vi "Close CurrentSource.vi"(6 "Source 2":T1(ring), 8 "error in (no error)":errorcluster, 10 "task in":refnum<k24>, 11 "VISA Refnum in":refnum<visa-resource-name>) -> ()   [LabVIEW 2024]
uses:
  <instrlib>/ULx/ULx_LV.dll
  Documents/LabVIEW Data/TestHarnessDPL_v24/Program Files/National Instruments/LabVIEW 2024/instr.lib/Keithley 24XX/Keithley 24XX.lvlib
panel:
  out "error out":errorcluster
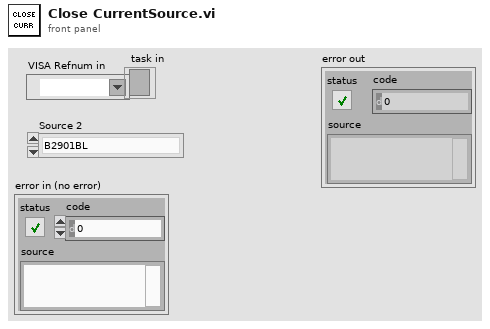
[diagram p1: front panel]
types:
  T1 = enum16{"B2901BL", "USB-3104 10M o/p3", "USB-3104 100K o/p5"}
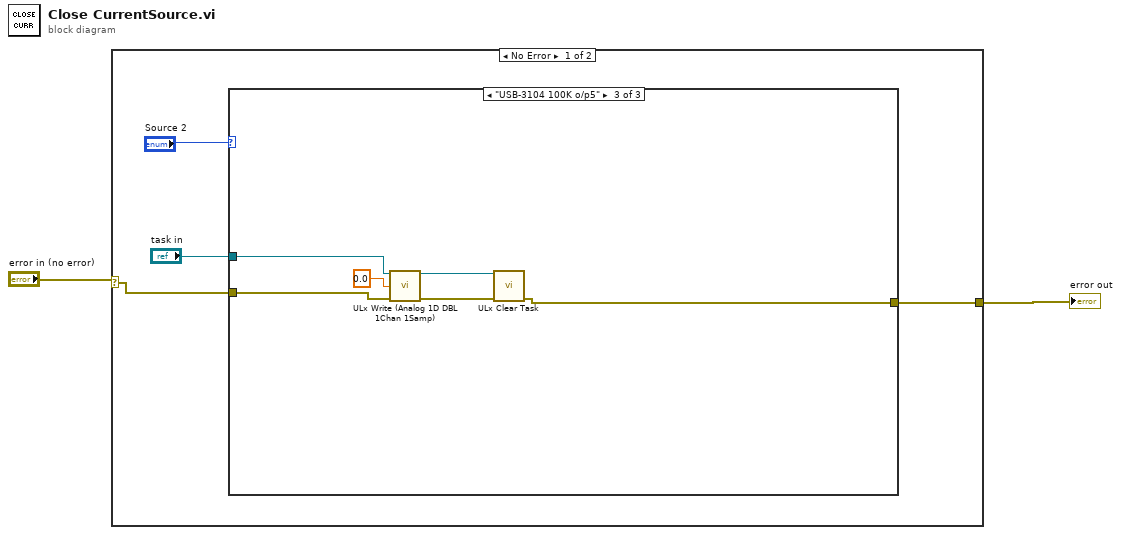
[diagram p0: block diagram]
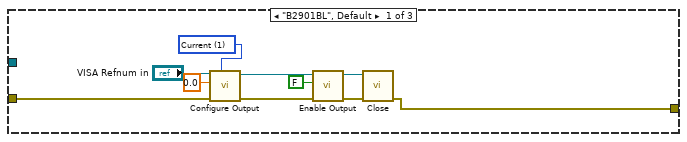
[diagram p2: hidden frame]
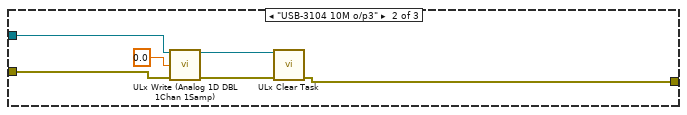
[diagram p3: hidden frame]
diagram:
  n1 = case shown="No Error" "error in (no error)" {
    selector: "error in (no error)" -> [w6 w29]
    tunnel: [w5 w29] -> w1
    frame No Error {
      n2 = case shown="\"USB-3104 100K o/p5\"" "Source 2" {
        tunnel: w6 -> [w8 w20 w26]
        tunnel: [w7 w22 w28] -> w5
        tunnel: "task in" -> [_ w17 w23]
        frame "B2901BL", Default {
          w11 = u16 1 items=["Voltage", "Current"] ("Source Mode  (0: Voltage)")
          n3 = call "Configure Output.vi"("Source Mode  (0: Voltage)"=w11, "error in (no error)"=w8, "Output Level (0)"=0.0, "VISA resource name"="VISA Refnum in") -> ("error out"=w12:errorcluster, "VISA resource name out"=w13:refnum<visa-resource-name>)  [unwired: 6 in]
          n4 = call "Enable Output.vi"("error in (no error)"=w12, "Enable Output (T: Enable)"=FALSE, "VISA resource name"=w13) -> ("error out"=w16:errorcluster, "VISA resource name out"=w15:refnum<visa-resource-name>)  [unwired: 7 in]
          n5 = call "Close.vi"("error in (no error)"=w16, "VISA resource name"=w15) -> ("error out"=w7:errorcluster)  [unwired: 9 in]
        }
        frame "USB-3104 10M o/p3" {
          n6 = call "ULx Write (Analog 1D DBL 1Chan 1Samp).vi"("task in"=w17, "data"=0.0, "error in"=w20) -> ("task out"=w19:refnum<k24>, "error out"=w21:errorcluster)  [unwired: 10 in, 1 out]
          n7 = call "ULx Clear Task.vi"("task in"=w19, "error in"=w21) -> ("error out"=w22:errorcluster)  [unwired: 13 in]
        }
        frame "USB-3104 100K o/p5" {
          n8 = call "ULx Write (Analog 1D DBL 1Chan 1Samp).vi"("task in"=w23, "data"=0.0, "error in"=w26) -> ("task out"=w25:refnum<k24>, "error out"=w27:errorcluster)  [unwired: 10 in, 1 out]
          n9 = call "ULx Clear Task.vi"("task in"=w25, "error in"=w27) -> ("error out"=w28:errorcluster)  [unwired: 13 in]
        }
      }
    }
    frame Error {
    }
  }
  "error out" <- w1
